vi "Fetch.vi"(0 "RS232 Port In":refnum<visa-resource-name>="COM1", 1 "Sensor Address In":string="a", 2 "Measurement Type In (Normal)":i32(ring) items=["Normal", "Concurrent", "Continuous"], 3 "Number of Measurements In (1)":i32=1, 5 "Error In (No Error)":errorcluster, 6 "CRC (False)":bool, 8 "Parameter In (0)":i32(ring) items=["0", "1", "2", "3", "4", "5", "6", "7", "8", "9"]) -> (10 "Parameter Out":i32(ring) items=["0", "1", "2", "3", "4", "5", "6", "7", "8", "9"], 12 "CRC Out":bool, 14 "RS232 Port Out":refnum<visa-resource-name>="COM1", 15 "Sensor Address Out":string="a", 16 "Measurement Type Out":i32(ring) items=["Normal", "Concurrent", "Continuous"], 17 "Number of Measurements Out":i32, 18 "Measurements Out":dbl[](array[numeric]), 19 "Error Out":errorcluster)   [LabVIEW 2016, in "SDI-12.lvlib"]
doc: "Fetches the data from a sensor. This VI may be called from any Measurement Type (Normal, Concurrent, Continuous)."
uses:
  SDI-12.lvlib
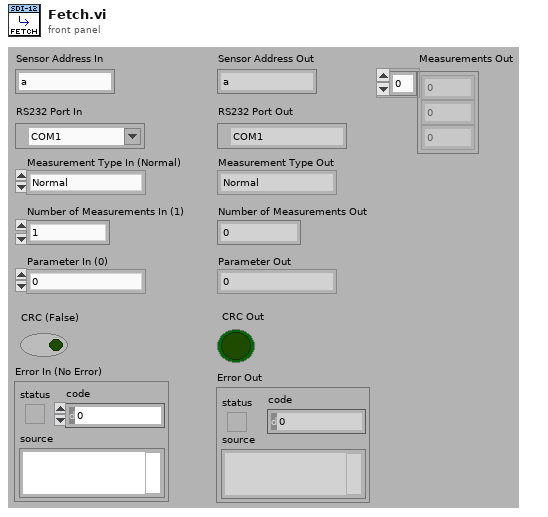
[diagram p1: front panel]
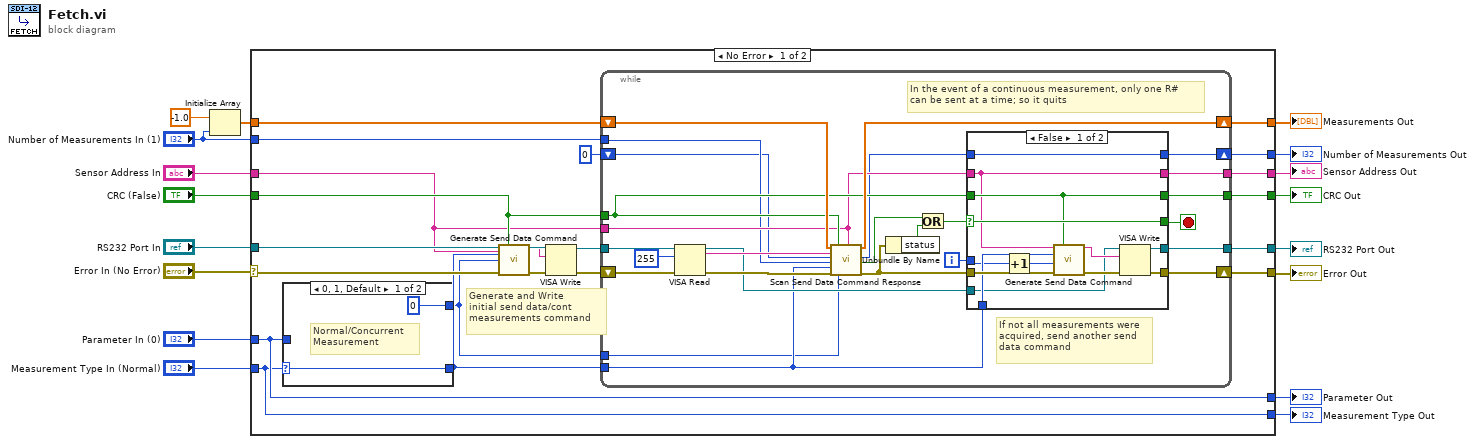
[diagram p0: block diagram]
diagram:
  n1 = Initialize Array(-1.0 ("Numeric"), "Number of Measurements In (1)") -> (w9:dbl[])
  n2 = case shown="No Error" "Error In (No Error)" {
    selector: "Error In (No Error)" -> [w34 w94]
    tunnel: [w27 w94] -> w17
    tunnel: [w28 w95] -> w16
    tunnel: "RS232 Port In" -> [w36 w95]
    tunnel: "Measurement Type In (Normal)" -> [w22 w91]
    tunnel: "Parameter In (0)" -> [w23 w92]
    tunnel: "Number of Measurements In (1)" -> [w29 w88]
    tunnel: "Sensor Address In" -> [w26 w89]
    tunnel: "CRC (False)" -> [w31 w90]
    tunnel: [w30 w93] -> w13
    tunnel: w9 -> [w24 w93]
    tunnel: [w23 w92] -> w5
    tunnel: [w22 w91] -> w4
    tunnel: [w21 w90] -> w3
    tunnel: [w20 w89] -> w2
    tunnel: [w18 w88] -> w1
    frame No Error {
      # "Generate and Write \ninitial send data/cont\nmeasurements command"
      n3 = case shown="0, 1, Default" w22 {
        selector: w22 -> [w39 w42]
        tunnel: [0 ("send iteration") w41] -> w25
        tunnel: [w39 w42] -> w33
        tunnel: w23 -> [_ w41]
        frame 0, 1, Default {
          # "Normal/Concurrent\nMeasurement"
        }
        frame 2 {
          # "Continuous mode:\nUse parameter to indentify\nwhich R# to generate"
        }
      }
      n4 = call "Generate Send Data Command.vi"("Sensor Address In"=w26, "CRC (False)"=w31, "Measurement Type In (Normal)"=w33, "Send Iteration (0)"=w25, "Error In (No Error)"=w34) -> ("Send Command"=w32:string, "Error Out"=w37:errorcluster)  [unwired: 9 in]
      n5 = VISA Write(VISA resource name=w36, write buffer=w32, error in (no error)=w37) -> (VISA resource name out=w38:refnum<visa-resource-name>, error out=w35:errorcluster)  [unwired: 1 out]
      n6 = while {
        tunnel: w38 -> [w66]
        shift-right: [w62] -> w30
        shift-left: w24 -> [w63]
        shift-right: [w58] -> w27
        shift-left: w35 -> [w61]
        tunnel: w33 -> [w52]
        tunnel: w31 -> [w60]
        tunnel: w26 -> [w51]
        tunnel: [w57] -> w28
        tunnel: w29 -> [w47]
        tunnel: w25 -> [w50]
        tunnel: [w49] -> w21
        tunnel: [w48] -> w20
        shift-right: [w45] -> w18
        shift-left: 0 ("Total Measurements Out") -> [w44]
        i -> [w64]
        stop <- w68 stop-if-true
        # "In the event of a continuous measurement, only one R#\ncan be sent at a time; so it quits"
        # "If not all measurements were\nacquired, send another send\ndata command"
        n7 = VISA Read(VISA resource name=w66, byte count=u32 255, error in (no error)=w61) -> (VISA resource name out=w56:refnum<visa-resource-name>, read buffer=w67:string, error out=w59:errorcluster)  [unwired: 1 out]
        n8 = call "Scan Send Data Command Response.vi"("Measurements In"=w63, "Sensor Response"=w67, "Total Measurements In"=w44, "Expected Measurements (1)"=w47, "Measurement Type In (Normal)"=w52, "Error In (No Error)"=w59, "CRC (False)"=w60, "Parameter In (0)"=w50, "Sensor Address In"=w51) -> ("Measurements Out"=w62:dbl[], "Total Measurements Out"=w46:i32, "Complete?"=w54:bool, "Error Out"=w55:errorcluster)  [unwired: 6 in, 1 out]
        n9 = Unbundle By Name(w55) -> ("status"=w43:bool)
        n10 = Or(x=w54, y=w43) -> (x .or. y?=w53:bool)
        n11 = case shown="False" w53 {
          selector: w53 -> [w81 w87]
          tunnel: [w81 w87] -> w68
          tunnel: w64 -> [w70 _]
          tunnel: w55 -> [w78 w86]
          tunnel: w51 -> [w72 w83]
          tunnel: w60 -> [w73 w84]
          tunnel: w52 -> [w77 _]
          tunnel: [w76 w85] -> w57
          tunnel: [w75 w86] -> w58
          tunnel: w56 -> [w74 w85]
          tunnel: [w73 w84] -> w49
          tunnel: [w72 w83] -> w48
          tunnel: w46 -> [w71 w82]
          tunnel: [w71 w82] -> w45
          frame False {
            n12 = Increment(x=w70) -> (x+1=w69:i32)
            n13 = call "Generate Send Data Command.vi"("Sensor Address In"=w72, "CRC (False)"=w73, "Measurement Type In (Normal)"=w77, "Send Iteration (0)"=w69, "Error In (No Error)"=w78) -> ("Send Command"=w79:string, "Error Out"=w80:errorcluster)  [unwired: 9 in]
            n14 = VISA Write(VISA resource name=w74, write buffer=w79, error in (no error)=w80) -> (VISA resource name out=w76:refnum<visa-resource-name>, error out=w75:errorcluster)  [unwired: 1 out]
          }
          frame True {
          }
        }
      }
    }
    frame Error {
    }
  }
  "Error Out" <- w17
  "RS232 Port Out" <- w16
  "Measurements Out" <- w13
  "Parameter Out" <- w5
  "Measurement Type Out" <- w4
  "Number of Measurements Out" <- w1
  "Sensor Address Out" <- w2
  "CRC Out" <- w3
